vi "CRYUpdate TS Structure.vi"(4 "Move Count":i32, 6 "Edit Step Num":i32, 7 "Tree Task SequenceIn":refnum<vi>, 8 "Target Index":i32, 9 "Count":i32, 10 "Source Index":i32, 11 "sOption":string) -> ()   [LabVIEW 2013]
uses:
  CRYProject Editor Global.vi
panel:
  out "Test Array Out":string[](array[string])
  in  "Test Array In":string[](array[string])
  in  "Move Up":bool
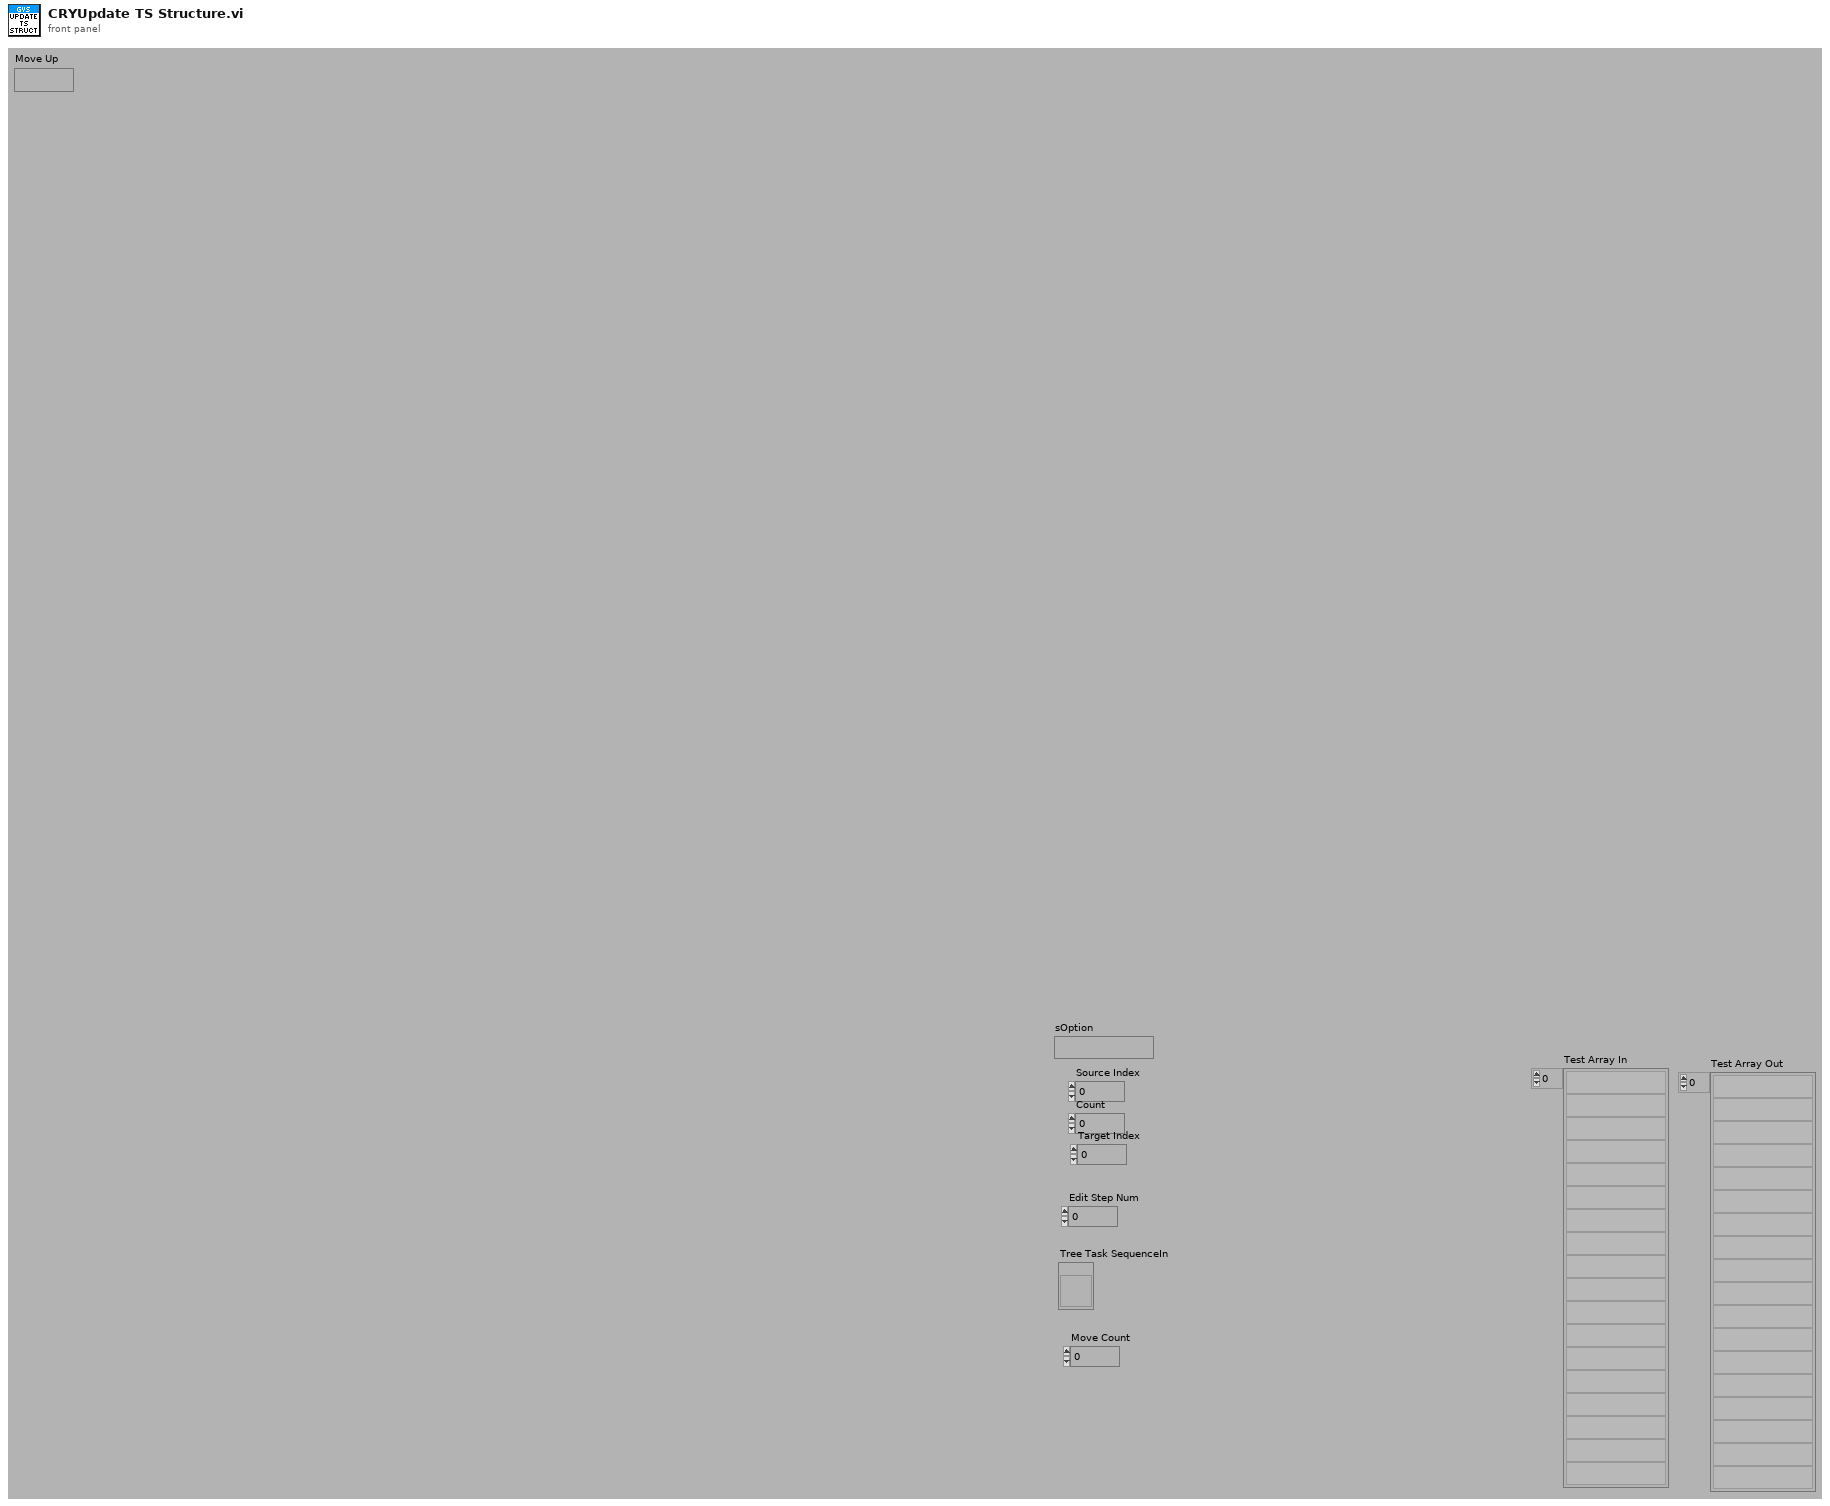
[diagram p1: front panel]
types:
  T1 = typedef "CRYTS.ctl" = cluster{"No.TS":u16, "TS File Path":path, "TS Name":string, "EditStepName":string, "Steps":T2[], "New State":bool, "Change State":bool, "Flattened CurveLib Data":string, "Document Data":string, "EditStepNo":u16, "Operator Start File":string, "Sequence Type":string, "Sequence Language":string}
  T2 = typedef "CRYStep.ctl" = cluster{"No.VI":i32, "Category":string, "StepName":string, "Seq setup flattened":string, "Comment":string, "Steps config.":bool[], "Jump config":i32[], "Start":dbl, "Increment":dbl, "Name":string, "Unit":string, "Y data":u16, "Y prefix":string, "Y dB ref":dbl, "Y unit":string, "Repeat State Array":cluster{"Start":dbl, "Increment":dbl, "Count":i32, "Num":i32}[]}
  T3 = enum16{"Curves", "Values", "Results", "WFM", "All"}
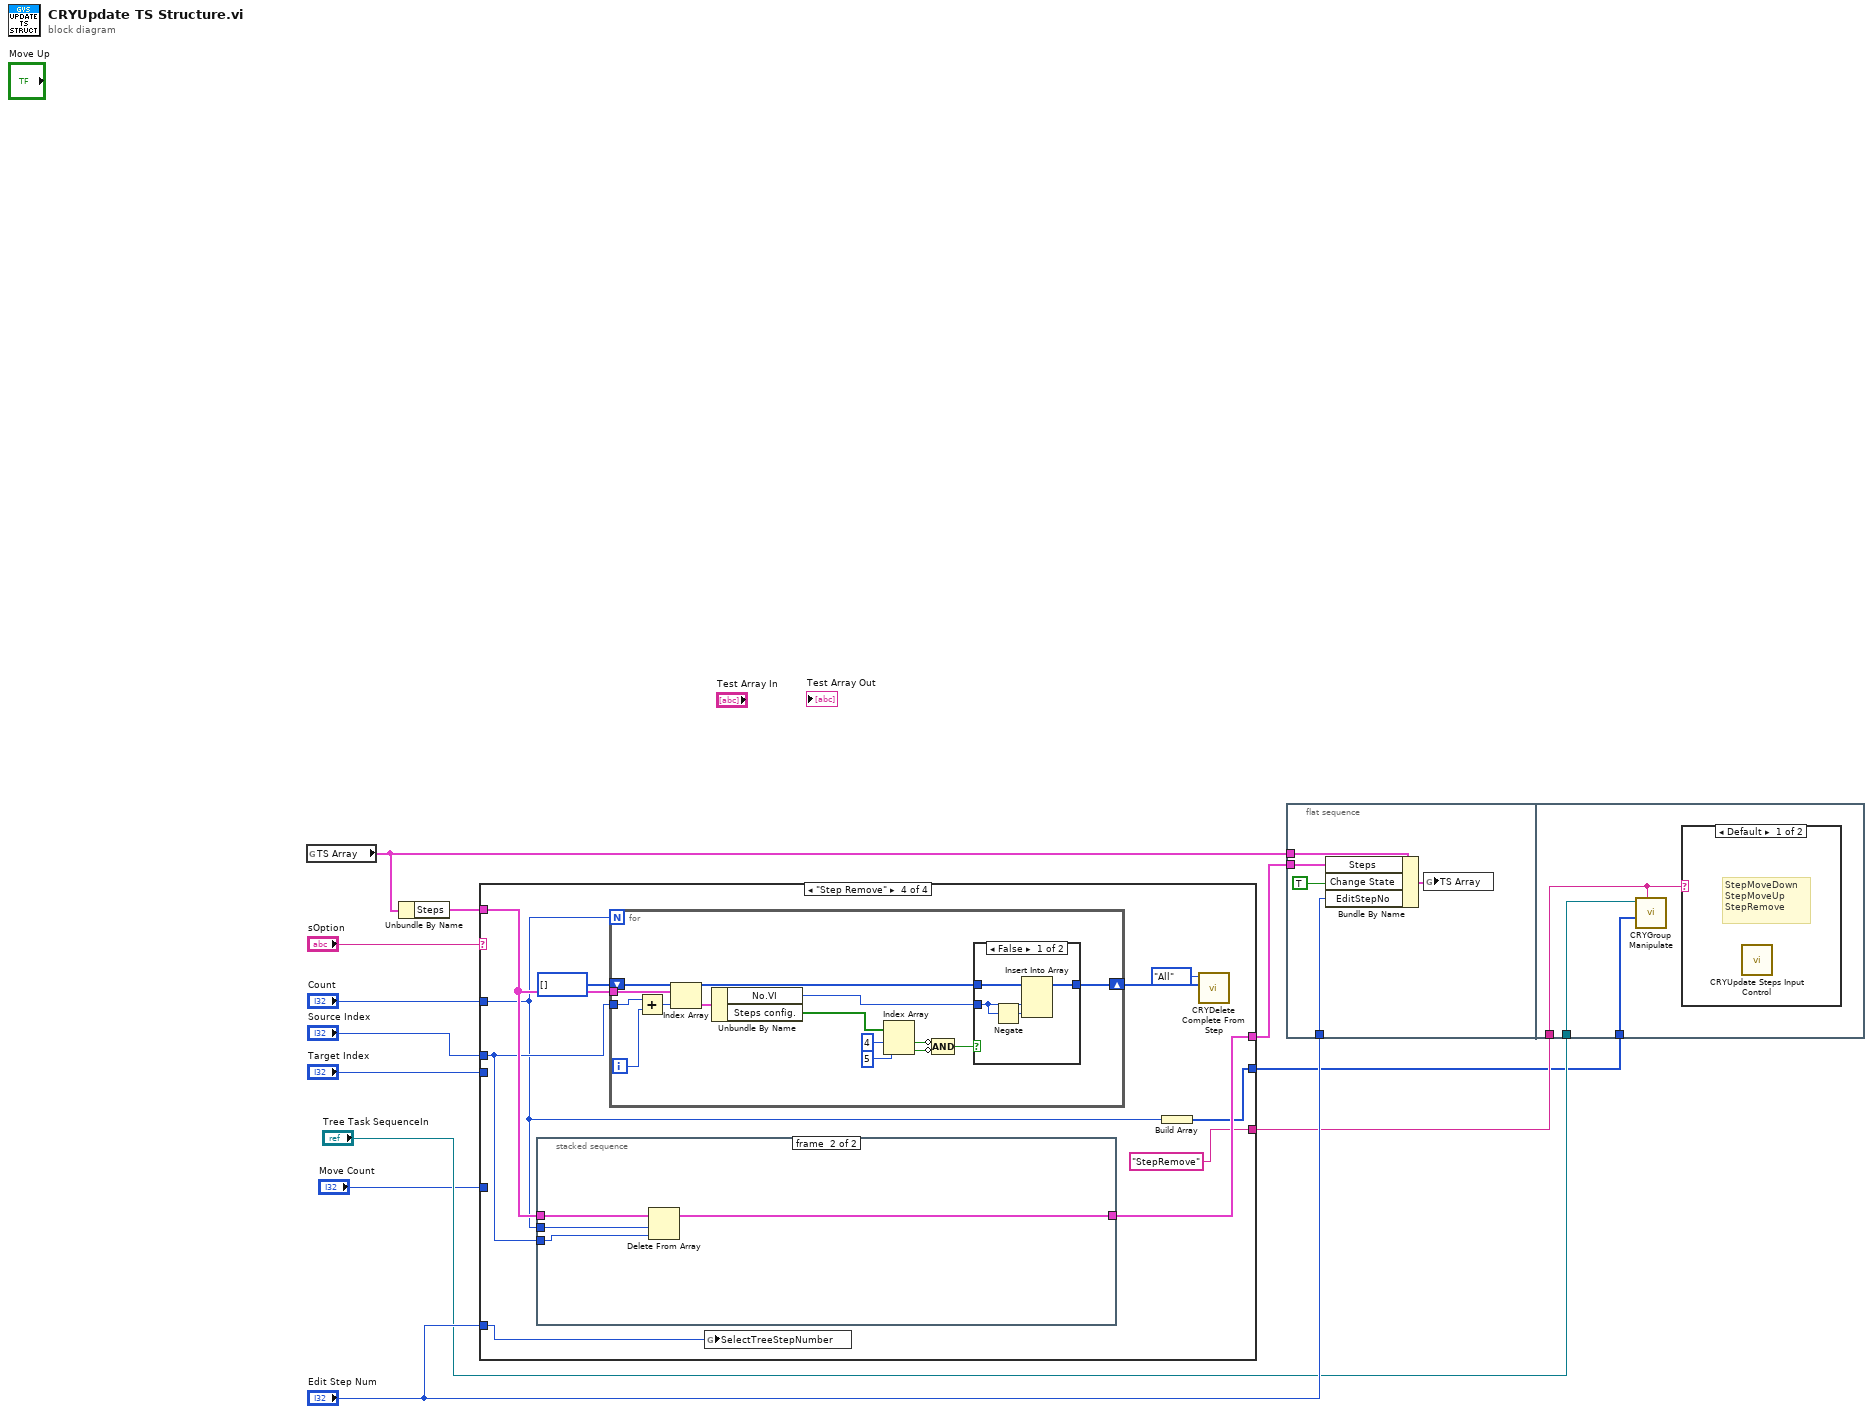
[diagram p0: block diagram]
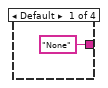
[diagram p3: hidden frame]
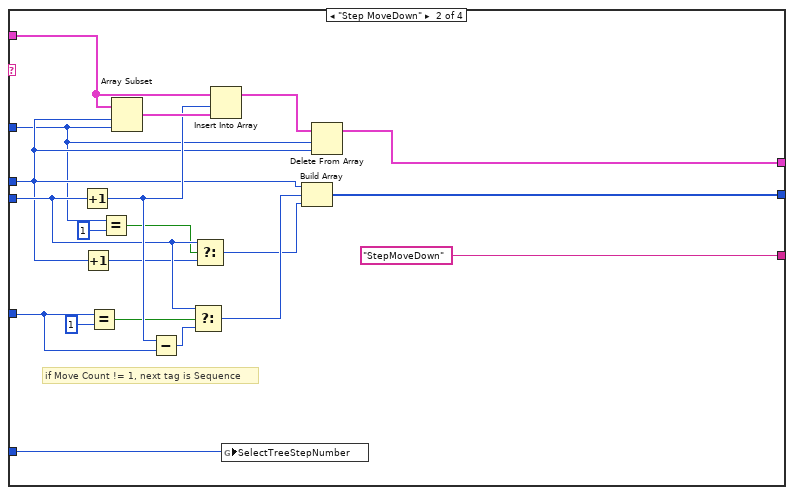
[diagram p4: hidden frame]
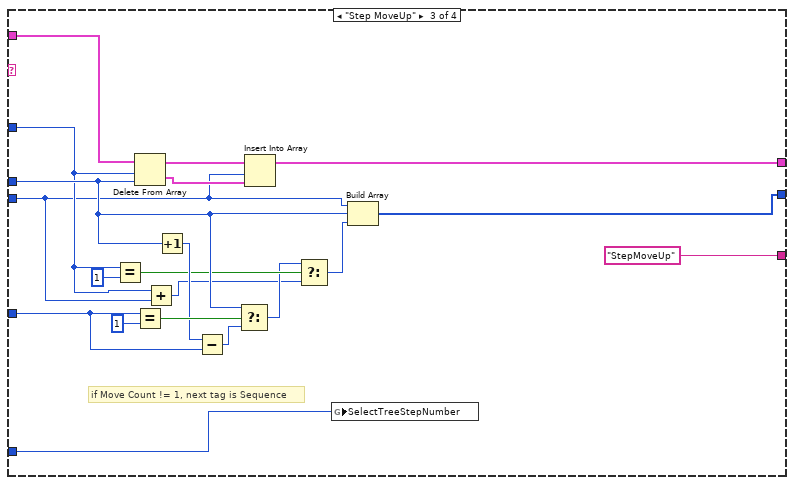
[diagram p5: hidden frame]
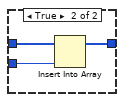
[diagram p6: hidden frame]
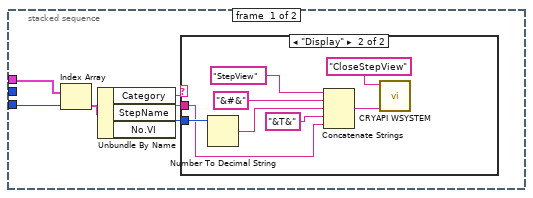
[diagram p7: hidden frame]
diagram:
  n1 = global read "CRYProject Editor Global.vi" "TS Array"() -> (w12:T1)
  n2 = Unbundle By Name(w12) -> ("Steps"=w8:T2[])
  n3 = case shown="\"Step Remove\"" "sOption" {
    tunnel: "Count" -> [_ w15 w36 w55]
    tunnel: "Source Index" -> [_ w18 w41 w59]
    tunnel: w8 -> [_ w31 w52 w62]
    tunnel: "Target Index" -> [_ w20 w34 _]
    tunnel: [_ w30 w51 w63] -> w7
    tunnel: ["None" ("sAction") "StepMoveDown" ("sAction") "StepMoveUp" ("sAction") "StepRemove" ("sAction")] -> w5
    tunnel: "Edit Step Num" -> [_ w28 w48 w56]
    tunnel: [_ w27 w43 w54] -> w2
    tunnel: "Move Count" -> [_ w25 w44 _]
    frame Default {
    }
    frame "Step MoveDown" {
      # "if Move Count != 1, next tag is Sequence"
      n4 = Increment(x=w20) -> (x+1=w22:i32)
      n5 = Increment(x=w18) -> (x+1=w17:i32)
      n6 = Equal?(x=w25, y=1) -> (x = y?=w21:bool)
      n7 = Equal?(x=w15, y=1) -> (x = y?=w14:bool)
      n8 = Array Subset(array=w31, index=w18, length=w15) -> (w33:T2[])
      n9 = Subtract(x=w22, y=w25) -> (x-y=w24:i32)
      n10 = Select(t=w20, s=w21, f=w24) -> (s? t:f=w23:i32)
      n11 = Select(t=w20, s=w14, f=w17) -> (s? t:f=w19:i32)
      n12 = Insert Into Array(array=w31, index=w22, new element=w33) -> (w32:T2[])
      n13 = global write "CRYProject Editor Global.vi" "SelectTreeStepNumber"(w28) -> ()
      n14 = Build Array(w18, w23, w19) -> (w27:i32[])
      n15 = Delete From Array(array=w32, length=w15, index=w18) -> (array with subset deleted=w30:T2[])  [unwired: 1 out]
    }
    frame "Step MoveUp" {
      # "if Move Count != 1, next tag is Sequence"
      n16 = Equal?(x=w36, y=1) -> (x = y?=w39:bool)
      n17 = Delete From Array(array=w52, length=w36, index=w41) -> (deleted portion=w53:T2[], array with subset deleted=w50:T2[])
      n18 = Equal?(x=w44, y=1) -> (x = y?=w45:bool)
      n19 = Add(x=w36, y=w34) -> (x+y=w35:i32)
      n20 = Increment(x=w41) -> (x+1=w42:i32)
      n21 = Subtract(x=w42, y=w44) -> (x-y=w46:i32)
      n22 = Select(t=w41, s=w45, f=w46) -> (s? t:f=w38:i32)
      n23 = Insert Into Array(array=w50, index=w34, new element=w53) -> (w51:T2[])
      n24 = Select(t=w38, s=w39, f=w35) -> (s? t:f=w37:i32)
      n25 = global write "CRYProject Editor Global.vi" "SelectTreeStepNumber"(w48) -> ()
      n26 = Build Array(w34, w41, w37) -> (w43:i32[])
    }
    frame "Step Remove" {
      n27 = stacked-sequence {
        tunnel: w59 -> [w87 w102]
        tunnel: w62 -> [w86 w101]
        tunnel: [_ w100] -> w63
        tunnel: w55 -> [_ w99]
        frame #0 {
          n28 = Index Array(array=w86, index=w87) -> (element=w90:T2)
          n29 = Unbundle By Name(w90) -> ("Category"=w89:string, "StepName"=w88:string, "No.VI"=w85:i32)
          n30 = case shown="\"Display\"" w89 {
            tunnel: w88 -> [_ w92]
            tunnel: w85 -> [_ w97]
            frame Default {
            }
            frame "Display" {
              n31 = Number To Decimal String(number=w97) -> (decimal integer string=w95:string)  [unwired: 1 in]
              n32 = Concatenate Strings("StepView" ("string"), "&#&" ("string"), w95, "&T&" ("string"), w92) -> (w96:string)
              n33 = call "CRYAPI WSYSTEM.vi"("sData"=w96, "sAction"="CloseStepView") -> ()  [unwired: 6 in, 4 out]
            }
          }
        }
        frame #1 {
          n34 = Delete From Array(array=w101, length=w99, index=w102) -> (array with subset deleted=w100:T2[])  [unwired: 1 out]
        }
      }
      n35 = for {
        N: w55 -> [_]
        tunnel: w59 -> [w74]
        tunnel: w62 -> [w76]
        shift-right: [w71] -> w60
        shift-left: i32[] [] -> [w72]
        i -> [w73]
        n36 = Add(x=w74, y=w73) -> (x+y=w75:i32)
        n37 = Index Array(array=w76, index=w75) -> (element=w77:T2)
        n38 = Unbundle By Name(w77) -> ("No.VI"=w70:i32, "Steps config."=w69:bool[])
        n39 = Index Array(array=w69, index #1=4 ("index"), index #2=5 ("index")) -> (element #1=w67:bool, element #2=w68:bool)
        n40 = Compound Arithmetic op=AND(invert w67, invert w68) -> (w64:bool)
        n41 = case shown="False" w64 {
          tunnel: w72 -> [w81 w84]
          tunnel: [w80 w83] -> w71
          tunnel: w70 -> [w79 w82]
          frame False {
            n42 = Negate(x=w79) -> (-x=w78:i32)
            n43 = Insert Into Array(array=w81, new element #1=w79, new element #2=w78) -> (w80:i32[])  [unwired: 1 in]
          }
          frame True {
            n44 = Insert Into Array(array=w84, new element=w82) -> (w83:i32[])  [unwired: 1 in]
          }
        }
      }
      n45 = global write "CRYProject Editor Global.vi" "SelectTreeStepNumber"(w56) -> ()
      n46 = Build Array(w55) -> (w54:i32[])
      n47 = call "CRYDelete Complete From Step.vi"("Step No."=w60, "Type In"=T3."All") -> ()  [unwired: 10 out]
    }
  }
  n48 = flat-sequence {
    tunnel: w12 -> [w106]
    tunnel: w7 -> [w104]
    tunnel: "Edit Step Num" -> [w103]
    tunnel: w5 -> [w109]
    tunnel: "Tree Task SequenceIn" -> [w110]
    tunnel: w2 -> [w108]
    frame #0 {
      n49 = Bundle By Name(cluster=w106, "Steps"=w104, "Change State"=TRUE, "EditStepNo"=w103) -> (w107:T1)
      n50 = global write "CRYProject Editor Global.vi" "TS Array"(w107) -> ()
    }
    frame #1 {
      n51 = call "CRYGroup Manipulate.vi"("sAction"=w109, "nData"=w108, "Tree in"=w110) -> ()  [unwired: 5 in, 4 out]
      n52 = case shown="Default" w109 {
        frame Default {
          # "StepMoveDown\nStepMoveUp\nStepRemove"
          n53 = call "CRYUpdate Steps Input Control.vi"() -> ()  [unwired: 12 in]
        }
        frame "None" {
        }
      }
    }
  }
